vi "tank drive final (default position button).vi"() -> ()   [LabVIEW 2010, in "Tank Robot.lvrbt"]
uses:
  Tank Robot.lvrbt
  <vilib>/NXT/Subs/LVHSConnector.ctl
  <vilib>/NXT/NXTIO Xnodes/AddressXNode/NXTIOAddress.xnode
  <vilib>/NXT/Subs/MotorXNode.Servo Type.ctl
  <vilib>/NXT/Subs/MotorXNode.1Servo.ctl
  <vilib>/NXT/NXTIO Xnodes/NXTIOXNode/NXTIO.xnode
  <vilib>/NXT/Subs/MotorXNode.DC Motor Type.ctl
  <vilib>/NXT/Subs/MotorXNode.2DCMotor.ctl
  <vilib>/NXT/NXTIO Xnodes/NXTIONodeSubVIs/TETRIX IO Move Servos.vi
  <vilib>/FTC/FTC Calculate Drive Power - Tank.vi
  <vilib>/NXT/NXTIO Xnodes/NXTIONodeSubVIs/TETRIX IO Move DC Motors.vi
  <vilib>/NXT/Dual Mode Library/Display/drawNumber_float.vi
panel:
  out "Numeric":dbl
  out "Default":bool
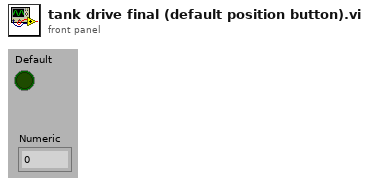
[diagram p1: front panel]
types:
  T1 = typedef "MotorXNode.Servo Type.ctl" = enum16{"Servo"}
  T2 = typedef "FTC ControllerState.ctl" = cluster{"Left X":i8, "Left Y":i8, "Right X":i8, "Right Y":i8, "Button Encoding 9-12":u8, "Button Encoding 1-8":u8, "POV":T3}
  T3 = typedef "FTC POVState.ctl" = i8
  T4 = typedef "FTC ButtonState.ctl" = cluster{"Button 1":bool, "Button 2":bool, "Button 3":bool, "Button 4":bool, "Button 5":bool, "Button 6":bool, "Button 7":bool, "Button 8":bool, "Button 9":bool, "Button 10":bool, "Button 11":bool, "Button 12":bool, "POV":T3}
  T5 = typedef "MotorXNode.DC Motor Type.ctl" = enum16{"DC Motor"}
  T6 = cluster{"DC Motor":T5, "Address":i16, "Address":i16}
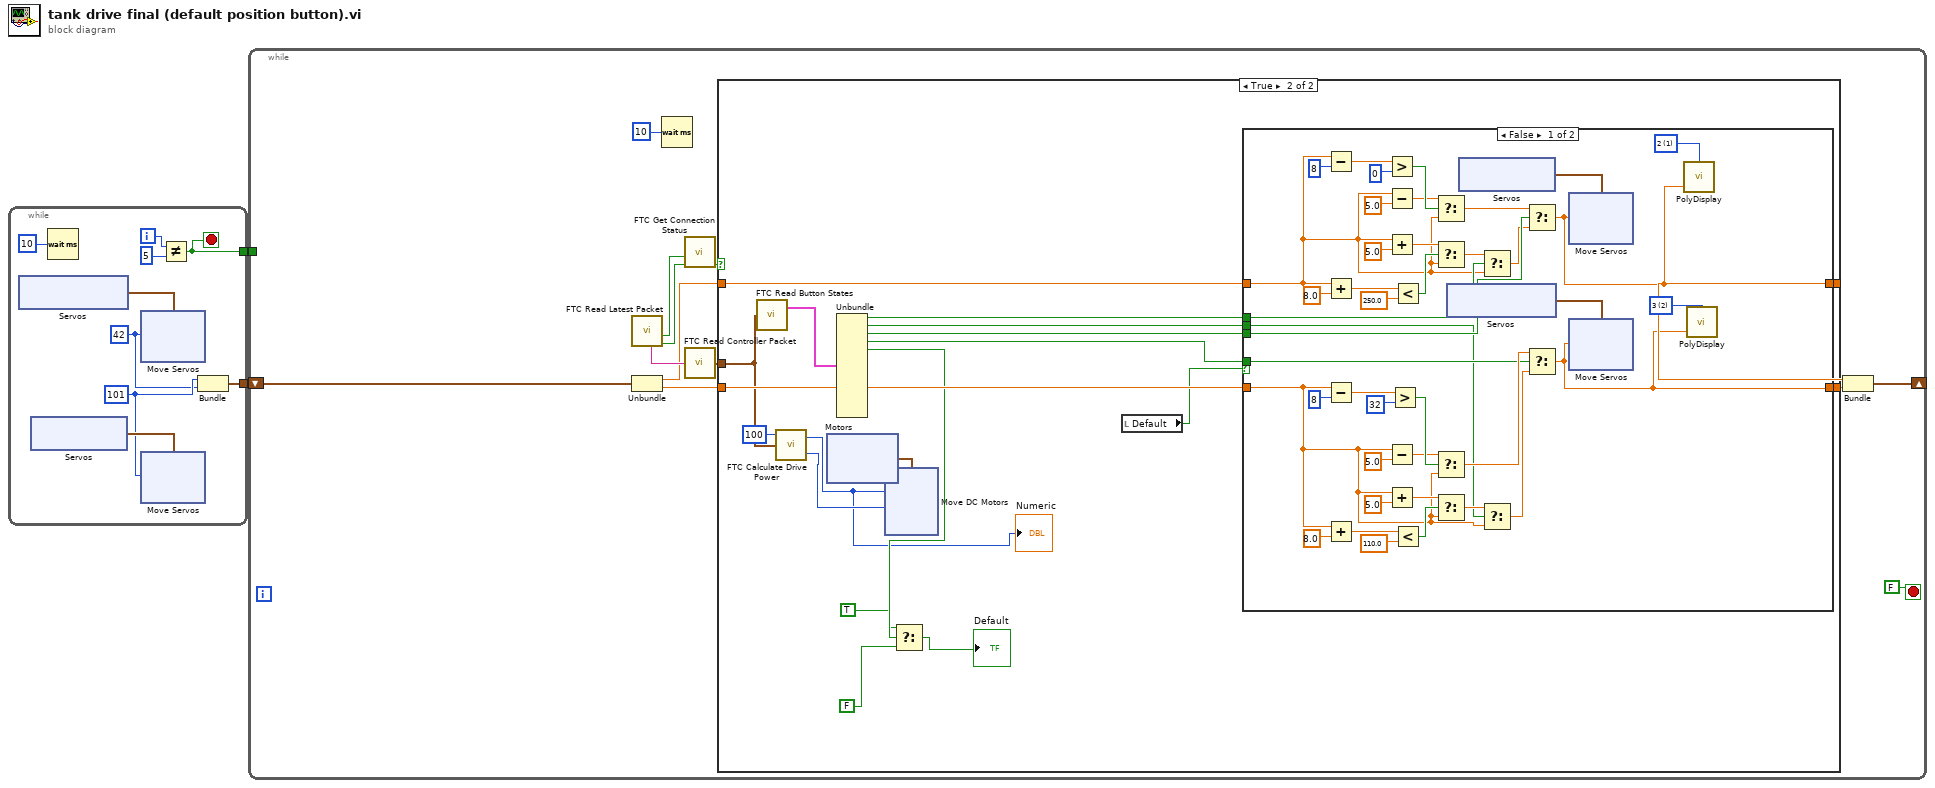
[diagram p0: block diagram]
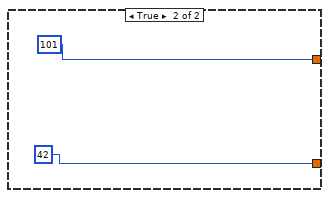
[diagram p3: hidden frame]
diagram:
  n1 = while {
    tunnel: [w8] -> w2
    tunnel: [w3] -> w1
    i -> [w11]
    stop <- w8 stop-if-true
    w4 = u8 42 ("Position 1")
    w5 = u8 101 ("Position 1")
    n2 = xnode "Servos"() -> ("Servo"=w6:cluster{"Servo":T1, "Address":i16})
    n3 = xnode "Servos"() -> ("Servo"=w7:cluster{"Servo":T1, "Address":i16})
    n4 = Wait (ms)(milliseconds to wait=u32 10) -> ()  [unwired: 1 out]
    n5 = xnode "Move Servos"("Position 1"=w4, "Servos"=w6) -> ()  [unwired: 1 in, 1 out]
    n6 = xnode "Move Servos"("Position 1"=w5, "Servos"=w7) -> ()  [unwired: 1 in, 1 out]
    n7 = Not Equal?(x=w11, y=5) -> (x != y?=w8:bool)
    n8 = Bundle("Position 1"=w5, "Position 1"=w4) -> (w3:cluster{"Position 1":u8, "Position 1":u8})  [unwired: 1 in]
  }
  n9 = while {
    tunnel: w2 -> [_]
    shift-right: [w30] -> _
    shift-left: w1 -> [w35]
    stop <- FALSE stop-if-true
    n10 = call <vilib>:"FTC Read Latest Packet.vi"() -> ("Packet Received?"=w39:bool, "Stopped?"=w40:bool, "Controller 1"=w37:string)  [unwired: 6 in, 3 out]
    n11 = Unbundle(w35) -> ("Position 1"=w34:dbl, "Position 1"=w33:dbl)
    n12 = Wait (ms)(milliseconds to wait=u32 10) -> ()  [unwired: 1 out]
    n13 = call <vilib>:"FTC Get Connection Status.vi"("Packet Received?"=w39, "Stopped?"=w40) -> ("Online?"=w38:bool)  [unwired: 6 in, 2 out]
    n14 = call <vilib>:"FTC Read Controller Packet.vi"("Packet"=w37) -> ("Controller State"=w36:T2)  [unwired: 4 in]
    n15 = case shown="True" w38 {
      tunnel: w36 -> [_ w55]
      tunnel: w34 -> [w44 w61]
      tunnel: w33 -> [w43 w57]
      tunnel: [w44 w60] -> w32
      tunnel: [w43 w56] -> w31
      frame False {
      }
      frame True {
        n16 = call <vilib>:"FTC Read Button States.vi"("Controller State"=w55) -> ("Button States"=w51:T4)  [unwired: 2 in, 1 out]
        n17 = call-poly <vilib>:"FTC Calculate Drive Power.vi"("Controller State"=w55, "Power Level (50)"=i8 100) -> ("Right Motor Power"=w52:i8, "Left Motor Power"=w45:i8)  [unwired: 2 in]
        "Numeric" <- w45
        n18 = xnode "Motors"() -> ("DC Motor"=w53:T6)
        n19 = Unbundle(w51) -> ("Button 1"=w62:bool, "Button 2"=w58:bool, "Button 3"=w63:bool, "Button 4"=w59:bool, "Button 5"=w50:bool)  [unwired: 8 out]
        n20 = xnode "Move DC Motors"("Power/Speed 2"=w52, "Power/Speed 1"=w45, "Motors"=w53) -> ()  [unwired: 1 in, 1 out]
        n21 = Select(t=TRUE, s=w50, f=FALSE) -> (s? t:f=→"Default":bool)
        n22 = local read "Default"() -> (w46:bool)
        n23 = case shown="False" w46 {
          tunnel: w63 -> [w97 _]
          tunnel: w62 -> [w96 _]
          tunnel: w61 -> [w88 _]
          tunnel: [w67 101] -> w60
          tunnel: w59 -> [w70 _]
          tunnel: w58 -> [w69 _]
          tunnel: w57 -> [w68 _]
          tunnel: [w65 42] -> w56
          frame False {
            w64 = i16 2 items=["1", "2", "3", "4", "5", "6", "7", "8"] ("Line")
            w66 = i16 1 items=["1", "2", "3", "4", "5", "6", "7", "8"] ("Line")
            n24 = Subtract(x=w88, y=u8 8) -> (x-y=w103:dbl)
            n25 = Add(x=w88, y=8.0) -> (x+y=w94:dbl)
            n26 = Subtract(x=w68, y=u8 8) -> (x-y=w84:dbl)
            n27 = Add(x=w68, y=8.0) -> (x+y=w77:dbl)
            n28 = Greater?(x=w103, y=u8 0) -> (0:w101:bool)
            n29 = Subtract(x=w88, y=5.0) -> (x-y=w100:dbl)
            n30 = Add(x=w88, y=5.0) -> (x+y=w91:dbl)
            n31 = Subtract(x=w68, y=5.0) -> (x-y=w81:dbl)
            n32 = Add(x=w68, y=5.0) -> (x+y=w74:dbl)
            n33 = Greater?(x=w84, y=u8 32) -> (0:w82:bool)
            n34 = Less?(x=w94, y=250.0) -> (x < y?=w92:bool)
            n35 = Less?(x=w77, y=110.0) -> (x < y?=w75:bool)
            n36 = Select(t=w100, s=w101, f=w88) -> (s? t:f=w98:dbl)
            n37 = Select(t=w91, s=w92, f=w88) -> (s? t:f=w89:dbl)
            n38 = Select(t=w81, s=w82, f=w68) -> (s? t:f=w79:dbl)
            n39 = Select(t=w74, s=w75, f=w68) -> (s? t:f=w72:dbl)
            n40 = xnode "Servos"() -> ("Servo"=w86:cluster{"Servo":T1, "Address":i16})
            n41 = xnode "Servos"() -> ("Servo"=w105:cluster{"Servo":T1, "Address":i16})
            n42 = Select(t=w89, s=w96, f=w88) -> (s? t:f=w87:dbl)
            n43 = Select(t=w72, s=w69, f=w68) -> (s? t:f=w71:dbl)
            n44 = Select(t=w98, s=w97, f=w87) -> (s? t:f=w67:dbl)
            n45 = Select(t=w79, s=w70, f=w71) -> (s? t:f=w65:dbl)
            n46 = xnode "Move Servos"("Position 1"=w67, "Servos"=w105) -> ()  [unwired: 1 in, 1 out]
            n47 = xnode "Move Servos"("Position 1"=w65, "Servos"=w86) -> ()  [unwired: 1 in, 1 out]
            n48 = call-poly <vilib>:"PolyDisplay.vi"("number"=w67, "Line"=w66) -> ()  [unwired: 2 in, 1 out]
            n49 = call-poly <vilib>:"PolyDisplay.vi"("number"=w65, "Line"=w64) -> ()  [unwired: 2 in, 1 out]
          }
          frame True {
          }
        }
      }
    }
    n50 = Bundle("Position 1"=w32, "Position 1"=w31) -> (w30:cluster{"Position 1":dbl, "Position 1":dbl})  [unwired: 1 in]
  }
